vi "writeToXML.vi"(8 "error in (no error)":errorcluster, 10 "Class Label":string, 11 "PointingPositions in":refnum<class "PointingPositions.lvclass">) -> (0 "error out":errorcluster, 2 "XML out":string, 3 "PointingPositions out":refnum<class "PointingPositions.lvclass">)   [LabVIEW 2014, in "TCSDataDefinitions.lvlib" / "TCSPublicStatus.lvlib" / "PointingPositions.lvlib" / "PointingPositions.lvclass"]
uses:
  PointingPositions.lvclass
  PointingPositions.lvclass/PointingPositions.ctl
  AzElError/AzElError.lvclass
  TCSCommand/TargetConfiguration/Target/FixedTarget/AzElParameters/AzElParameters.lvclass
  CurrentTimes/ClockTimes/ClockTimes.lvclass
  TCSCommand/TargetConfiguration/Target/FixedTarget/RADecParameters/RADecParameters.lvclass
  CurrentRotatorPositions/CurrentRotatorPositions.lvclass
  DifftrackStatus/DifftrackStatus.lvclass
  ObjectPA/ObjectPA.lvclass
  RotatorPositions/RotatorPositions.lvclass
  <userlib>/Common/XML/XMLGenerator/XMLGenerator.lvclass
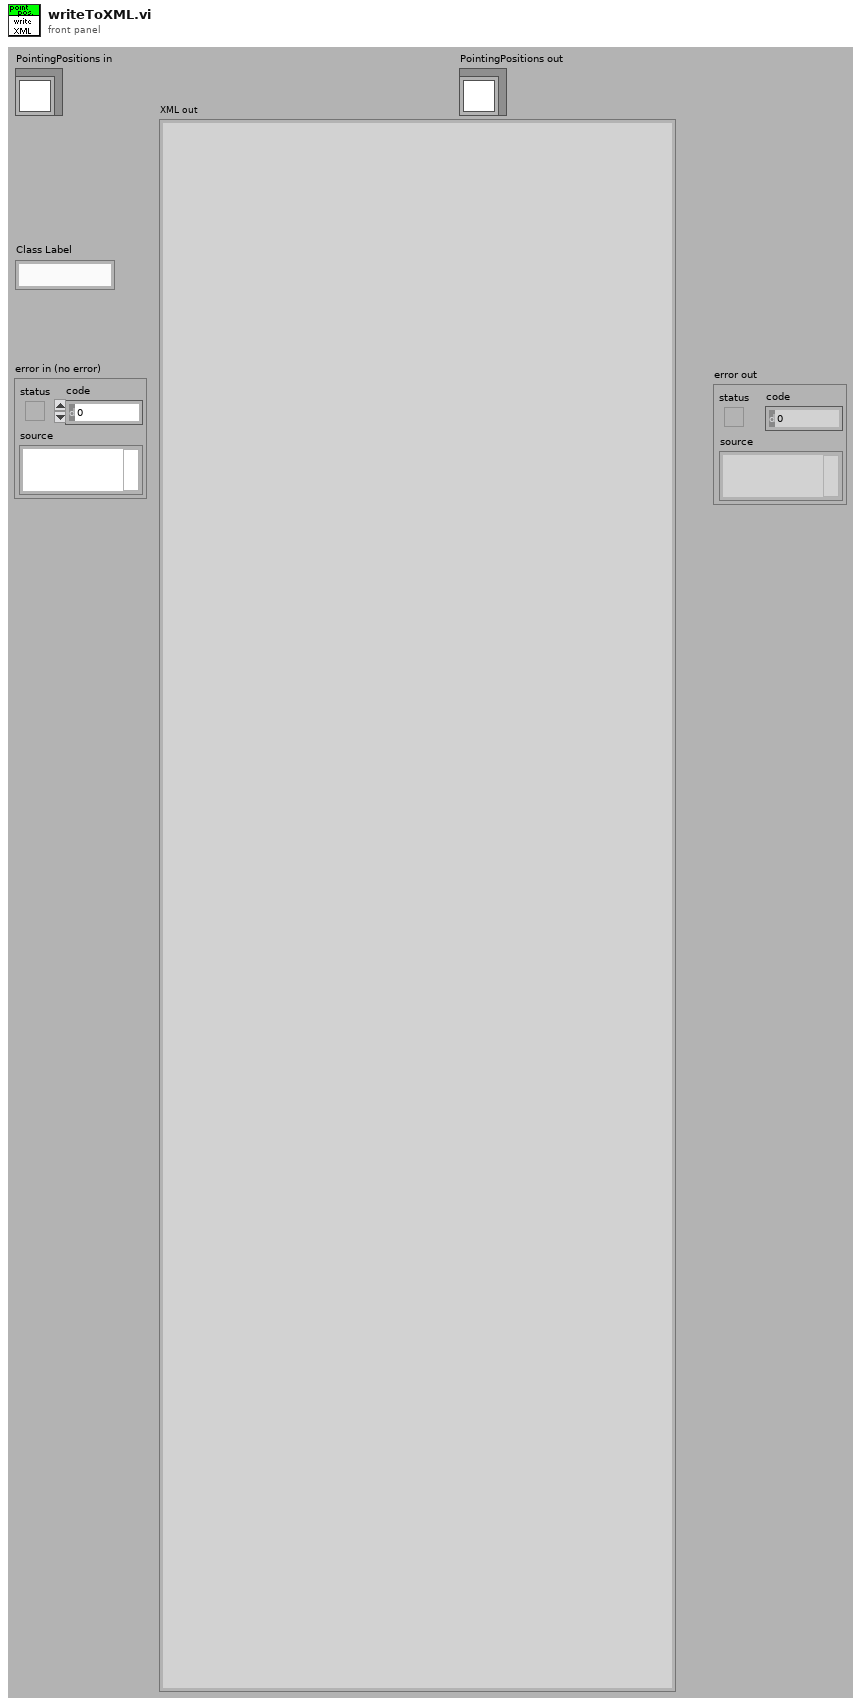
[diagram p1: front panel]
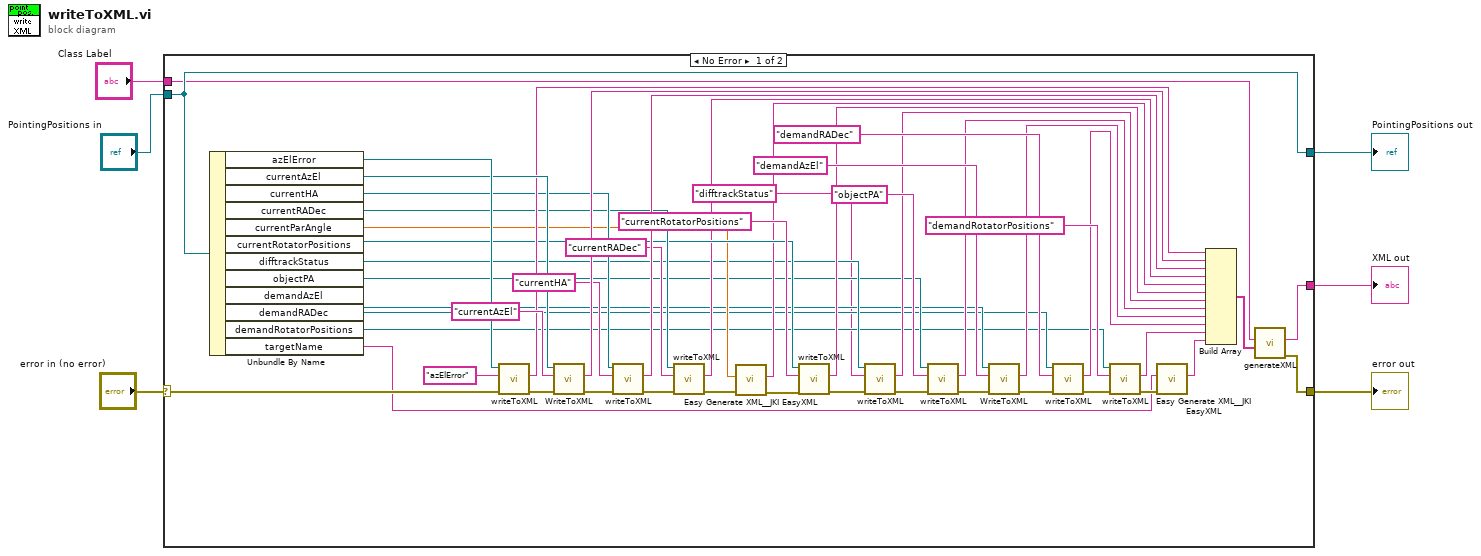
[diagram p0: block diagram]
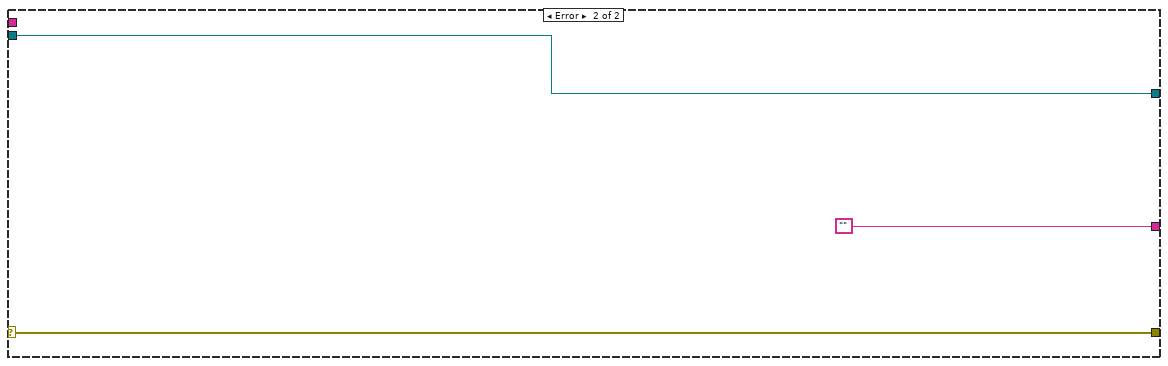
[diagram p2: hidden frame]
diagram:
  n1 = case shown="No Error" "error in (no error)" {
    selector: "error in (no error)" -> [w54 w60]
    tunnel: [w33 w60] -> w5
    tunnel: [w57 w59] -> w3
    tunnel: "PointingPositions in" -> [w57 w59]
    tunnel: [w34 ""] -> w2
    tunnel: "Class Label" -> [w31 _]
    frame No Error {
      n2 = Unbundle By Name(w57) -> ("azElError"=w56:refnum<class "AzElError.lvclass">, "currentAzEl"=w53:refnum<class "AzElParameters.lvclass">, "currentHA"=w48:refnum<class "ClockTimes.lvclass">, "currentRADec"=w43:refnum<class "RADecParameters.lvclass">, "currentParAngle"=w27:dbl, "currentRotatorPositions"=w30:refnum<class "CurrentRotatorPositions.lvclass">, "difftrackStatus"=w12:refnum<class "DifftrackStatus.lvclass">, "objectPA"=w11:refnum<class "ObjectPA.lvclass">, "demandAzEl"=w10:refnum<class "AzElParameters.lvclass">, "demandRADec"=w9:refnum<class "RADecParameters.lvclass">, "demandRotatorPositions"=w8:refnum<class "RotatorPositions.lvclass">, "targetName"=w21:string)
      n3 = call-dynamic "writeToXML.vi"("error in (no error)"=w54, "Class Label"="azElError", "AzElError in"=w56) -> ("error out"=w51:errorcluster, "XML out"=w50:string)  [unwired: 6 in, 1 out]
      n4 = call-dynamic "WriteToXML.vi"("error in (no error)"=w51, "Class Label"="currentAzEl", "AzElParameters in"=w53) -> ("error out"=w45:errorcluster, "XML out"=w49:string)  [unwired: 6 in, 1 out]
      n5 = call-dynamic "writeToXML.vi"("error in (no error)"=w45, "Class Label"="currentHA", "ClockTimes in"=w48) -> ("error out"=w42:errorcluster, "XML out"=w46:string)  [unwired: 6 in, 1 out]
      n6 = call-dynamic "writeToXML.vi"("error in (no error)"=w42, "Class Label"="currentRADec", "RADecParameters in"=w43) -> ("error out"=w28:errorcluster, "XML out"=w22:string)  [unwired: 6 in, 1 out]
      n7 = call <vilib>:"Easy Generate XML__JKI EasyXML.vi"("error in (no error)"=w28, "LabVIEW Data"=w27) -> ("error out"=w29:errorcluster, "XML String"=w26:string)  [unwired: 8 in]
      n8 = call-dynamic "writeToXML.vi"("error in (no error)"=w29, "Class Label"="currentRotatorPositions", "CurrentRotatorPositions in"=w30) -> ("error out"=w15:errorcluster, "XML out"=w23:string)  [unwired: 6 in, 1 out]
      n9 = call-dynamic "writeToXML.vi"("error in (no error)"=w15, "ClassLabel"="difftrackStatus" ("Class Label"), "DifftrackStatus in"=w12) -> ("error out"=w14:errorcluster, "XML out"=w13:string)  [unwired: 6 in, 1 out]
      n10 = call-dynamic "writeToXML.vi"("error in (no error)"=w14, "Class Label"="objectPA", "ObjectPA in"=w11) -> ("error out"=w25:errorcluster, "XML out"=w16:string)  [unwired: 6 in, 1 out]
      n11 = call-dynamic "WriteToXML.vi"("error in (no error)"=w25, "Class Label"="demandAzEl", "AzElParameters in"=w10) -> ("error out"=w38:errorcluster, "XML out"=w17:string)  [unwired: 6 in, 1 out]
      n12 = call-dynamic "writeToXML.vi"("error in (no error)"=w38, "Class Label"="demandRADec", "RADecParameters in"=w9) -> ("error out"=w36:errorcluster, "XML out"=w18:string)  [unwired: 6 in, 1 out]
      n13 = call-dynamic "writeToXML.vi"("error in (no error)"=w36, "Class Label"="demandRotatorPositions", "RotatorPositions in"=w8) -> ("error out"=w32:errorcluster, "XML out"=w19:string)  [unwired: 6 in, 1 out]
      n14 = call <vilib>:"Easy Generate XML__JKI EasyXML.vi"("error in (no error)"=w32, "LabVIEW Data"=w21) -> ("XML String"=w20:string)  [unwired: 8 in, 1 out]
      n15 = Build Array(w50, w49, w46, w22, w26, w23, w13, w16, w17, w18, w19, w20) -> (w35:string[])
      n16 = call <userlib>:"generateXML.vi"("childrenXML"=w35, "elementName"=w31) -> ("error out"=w33:errorcluster, "XML out"=w34:string)  [unwired: 7 in, 1 out]
    }
    frame Error {
    }
  }
  "error out" <- w5
  "PointingPositions out" <- w3
  "XML out" <- w2
